vi "MongoDB.FindOneByQuery.vi"(8 "error in (no error)":errorcluster, 10 "JSON Query String":string, 11 "MongoDB.Collection in":refnum<class "MongoDB.Collection.lvclass">) -> (0 "error out":errorcluster, 2 "Result":string, 3 "MongoDB.Collection out":refnum<class "MongoDB.Collection.lvclass">)   [LabVIEW 2014, in "MongoDB.Collection.lvclass"]
uses:
  MongoDB.Collection.lvclass
  MongoDB.Collection.lvclass/MongoDB.Collection.ctl
  C:/Users/Richard/Documents/GitHub/mongo-labview-driver/CSharp/bin/MongoDB.Driver.Legacy.dll
  CSharp/bin/MongoDB.Driver.Legacy.dll
  C:/Users/Richard/Documents/GitHub/mongo-labview-driver/CSharp/bin/MongoDB.Bson.dll
  CSharp/bin/MongoDB.Bson.dll
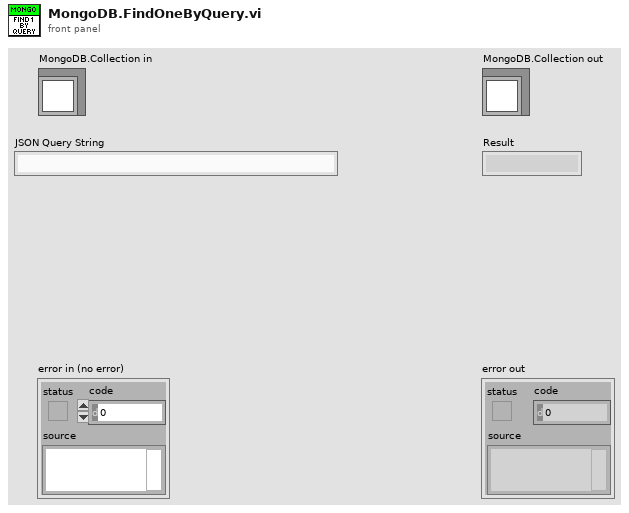
[diagram p1: front panel]
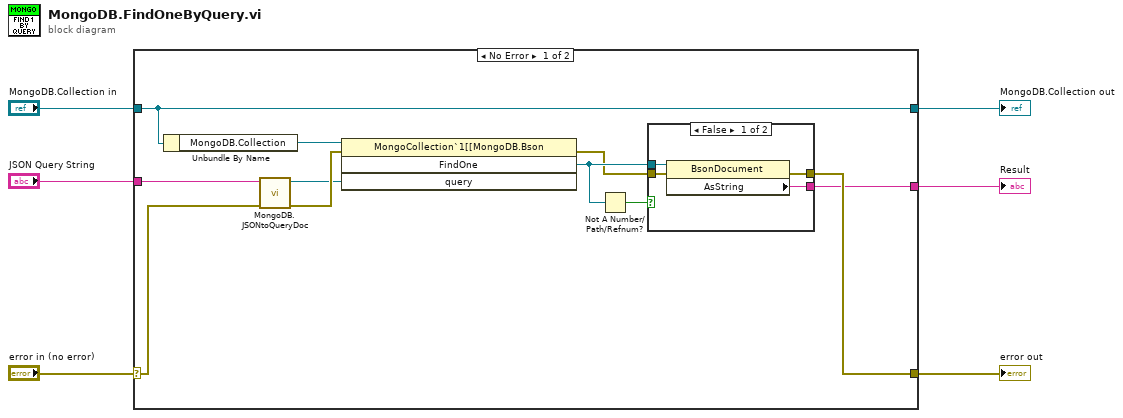
[diagram p0: block diagram]
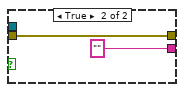
[diagram p2: hidden frame]
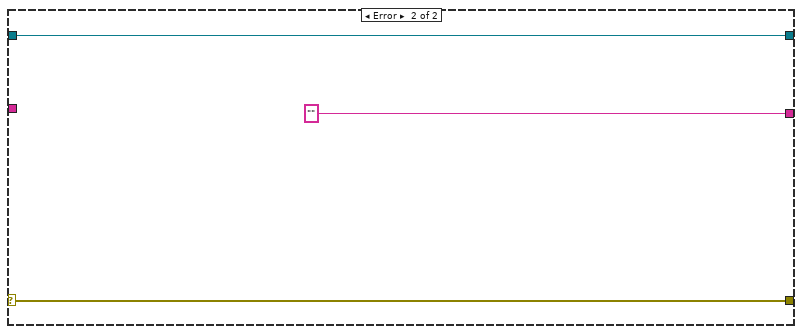
[diagram p3: hidden frame]
diagram:
  n1 = case shown="No Error" "error in (no error)" {
    selector: "error in (no error)" -> [w13 w26]
    tunnel: [w9 w26] -> w5
    tunnel: [w17 w25] -> w3
    tunnel: "MongoDB.Collection in" -> [w17 w25]
    tunnel: "JSON Query String" -> [w15 _]
    tunnel: [w8 "" ("ToString")] -> w1
    frame No Error {
      n2 = Unbundle By Name(w17) -> ("MongoDB.Collection"=w16:refnum<k24>)
      n3 = call "MongoDB.JSONtoQueryDoc.vi"("error in (no error)"=w13, "JSON Query String"=w15) -> ("error out"=w14:errorcluster, ".NET Refnum out"=w7:refnum<k24>)  [unwired: 8 in]
      n4 = invoke class="MongoCollection`1[[MongoDB.Bson" method="FindOne"(reference=w16, error in=w14, "query"=w7) -> (error out=w10:errorcluster, "FindOne"=w11:refnum<k24>)  [unwired: 1 in, 2 out]
      n5 = Not A Number/Path/Refnum?(number/path/refnum=w11) -> (NaN/Path/Refnum?=w12:bool)
      n6 = case shown="False" w12 {
        tunnel: [w21 "" ("AsString")] -> w8
        tunnel: w11 -> [w20 _]
        tunnel: w10 -> [w19 w22]
        tunnel: [w18 w22] -> w9
        frame False {
          n7 = property class="BsonDocument"(reference=w20, error in=w19) -> (error out=w18:errorcluster, "AsString"=w21:string)  [unwired: 1 out]
        }
        frame True {
        }
      }
    }
    frame Error {
    }
  }
  "error out" <- w5
  "MongoDB.Collection out" <- w3
  "Result" <- w1
